vi "Helper SubVI - System Mode Simulation.vi"(11 "mode num":i32=30) -> (2 "fault mode":dbl[][](array[numeric]), 3 "normal mode":dbl[][](array[numeric]))   [LabVIEW 2023]
doc: "Simulates normal and fault system modes."
uses:
  <vilib>/Analysis/3filter.llb/IIR Filter (DBL).vi
  <vilib>/Analysis/NI_AALBase.lvlib
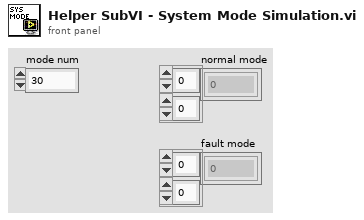
[diagram p1: front panel]
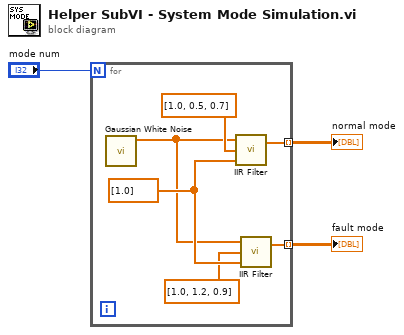
[diagram p0: block diagram]
diagram:
  n1 = for {
    N: "mode num" -> [_]
    tunnel: [w8] -> w1 mode=indexing
    tunnel: [w4] -> w2 mode=indexing
    w7 = dbl[] [1.0] ("Forward Coefficients")
    n2 = call <vilib>:"Gaussian White Noise.vi"() -> ("Gaussian noise pattern"=w5:dbl[])  [unwired: 10 in, 1 out]
    n3 = call-poly <vilib>:"IIR Filter.vi"("Forward Coefficients"=w7, "Reverse Coefficients"=dbl[] [1.0, 0.5, 0.7], "X"=w5) -> ("Filtered X"=w8:dbl[])  [unwired: 1 in, 1 out]
    n4 = call-poly <vilib>:"IIR Filter.vi"("Forward Coefficients"=w7, "Reverse Coefficients"=dbl[] [1.0, 1.2, 0.9], "X"=w5) -> ("Filtered X"=w4:dbl[])  [unwired: 1 in, 1 out]
  }
  "fault mode" <- w2
  "normal mode" <- w1
